vi "From Mapped Paths.vi"(0 "Paths":path[](array[path]), 1 "Key":string) -> (2 "Array":refnum<class "Array.lvclass">)   [LabVIEW 2018, in "Toolkit.lvlib" / "Data.lvlib" / "Array.lvclass"]
uses:
  Array.lvclass
  Array.lvclass/Array.ctl
  Map/Map.lvclass
  D:/Users/cfield/Code/Field R&D Services/Labstache/src/Toolkit/Data/Datum/Datum.lvclass
  Map/Support/From Path.vi
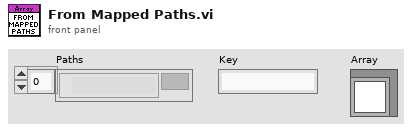
[diagram p1: front panel]
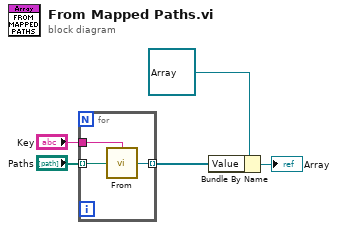
[diagram p0: block diagram]
diagram:
  n1 = for {
    tunnel: "Paths" -> [w8] mode=indexing
    tunnel: "Key" -> [w7]
    tunnel: [w6] -> w1 mode=indexing
    n2 = call-poly "From.vi"("Value"=w8, "Key"=w7) -> ("Map"=w6:refnum<class "Map.lvclass">)
  }
  n3 = Bundle By Name(cluster=refnum<class "Array.lvclass"> refnum ("Toolkit.lvlib:Data.lvlib:Array.lvclass"), "Value"=w1) -> (→"Array":refnum<class "Array.lvclass">)
